vi "Perform_AFP.vi"(8 "AFP Target":i32, 9 "rho-":dbl[](array[numeric]), 10 "rho0":dbl[](array[numeric]), 11 "rho+":dbl[](array[numeric])) -> (1 "rho- out":dbl[](array[numeric]), 2 "rho0 out":dbl[](array[numeric]), 3 "rho+ out":dbl[](array[numeric]))   [LabVIEW 2018]
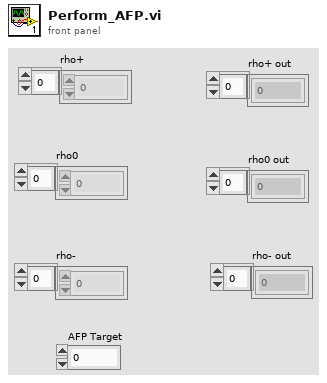
[diagram p1: front panel]
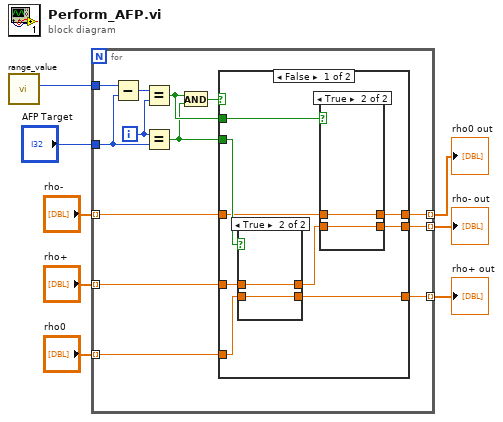
[diagram p0: block diagram]
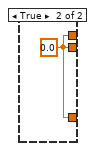
[diagram p4: hidden frame]
diagram:
  n1 = call "range_value.vi"() -> ("NumBins"=w1:i32)  [unwired: 10 in, 1 out]
  n2 = for {
    tunnel: "rho+" -> [w14] mode=indexing
    tunnel: "rho0" -> [w13] mode=indexing
    tunnel: "rho-" -> [w12] mode=indexing
    tunnel: w1 -> [w21]
    tunnel: "AFP Target" -> [w18]
    tunnel: [w11] -> w4 mode=indexing
    tunnel: [w10] -> w3 mode=indexing
    tunnel: [w9] -> w2 mode=indexing
    i -> [w19]
    n3 = Subtract(x=w21, y=w18) -> (x-y=w20:i32)
    n4 = Equal?(x=w20, y=w19) -> (x = y?=w17:bool)
    n5 = Equal?(x=w19, y=w18) -> (x = y?=w15:bool)
    n6 = And(x=w17, y=w15) -> (x .and. y?=w16:bool)
    n7 = case shown="False" w16 {
      tunnel: w17 -> [w30 _]
      tunnel: w15 -> [w29 _]
      tunnel: w14 -> [w28 _]
      tunnel: w13 -> [w27 _]
      tunnel: [w25 w39] -> w11
      tunnel: w12 -> [w24 _]
      tunnel: [w23 w39] -> w9
      tunnel: [w22 w39] -> w10
      frame False {
        n8 = case shown="True" w29 {
          tunnel: w28 -> [w32 w34]
          tunnel: w27 -> [w31 w33]
          tunnel: [w32 w33] -> w25
          tunnel: [w31 w34] -> w26
          frame False {
          }
          frame True {
          }
        }
        n9 = case shown="True" w30 {
          tunnel: w26 -> [w36 w38]
          tunnel: [w36 w37] -> w22
          tunnel: w24 -> [w35 w37]
          tunnel: [w35 w38] -> w23
          frame False {
          }
          frame True {
          }
        }
      }
      frame True {
        w39 = 0.0
      }
    }
  }
  "rho+ out" <- w4
  "rho0 out" <- w3
  "rho- out" <- w2
